vi "Parse Response for Result or Error.vi"(8 "error in":errorcluster, 10 "Response String In":string) -> (0 "error out":errorcluster, 1 "LabVIEW Error?":bool=TRUE, 2 "JSON Value out":variant)   [LabVIEW 2020, in "JSON-RPC Lib.lvlib" / "JSONRPC Client.lvclass"]
uses:
  JSONRPC Client.lvclass
  Variant JSON API/Variant JSON API.lvlib
  Variant Data Manipulation/Variant Data Manipulation.lvlib
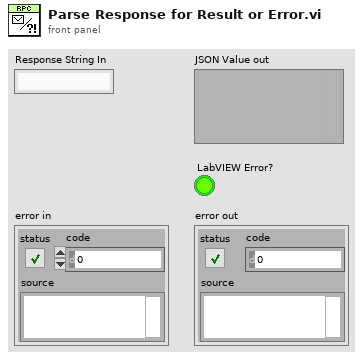
[diagram p1: front panel]
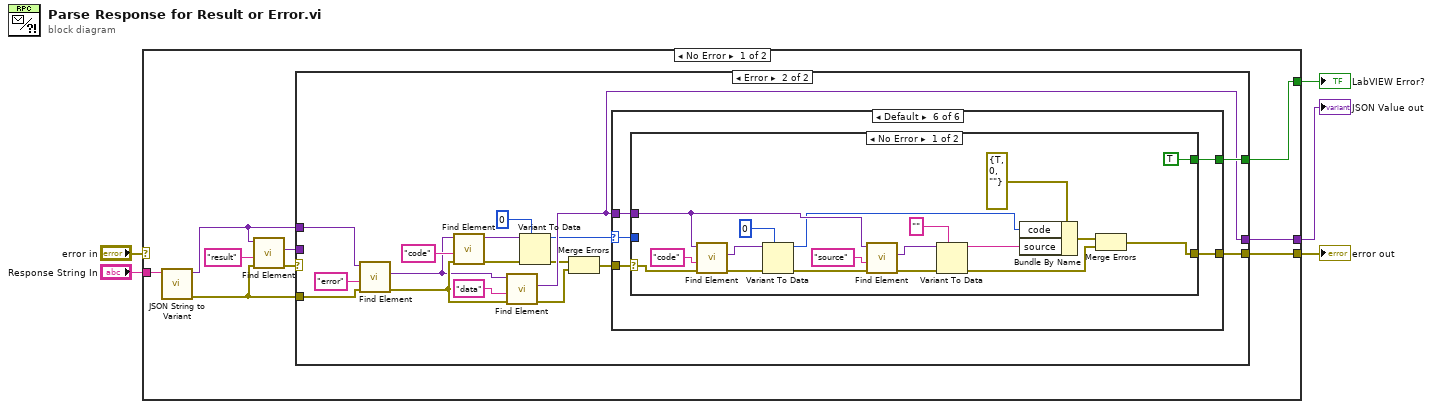
[diagram p0: block diagram]
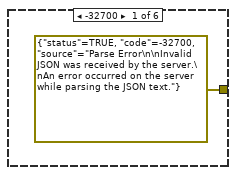
[diagram p3: hidden frame]
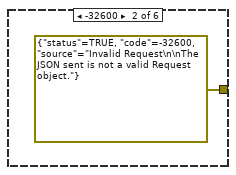
[diagram p4: hidden frame]
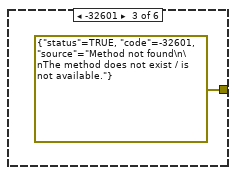
[diagram p5: hidden frame]
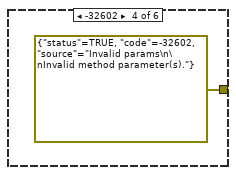
[diagram p6: hidden frame]
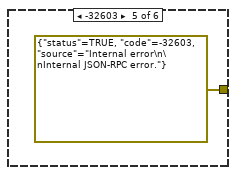
[diagram p7: hidden frame]
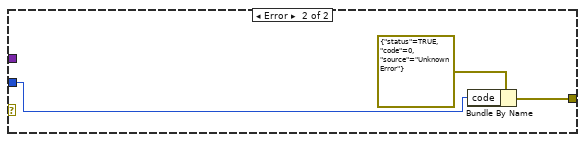
[diagram p8: hidden frame]
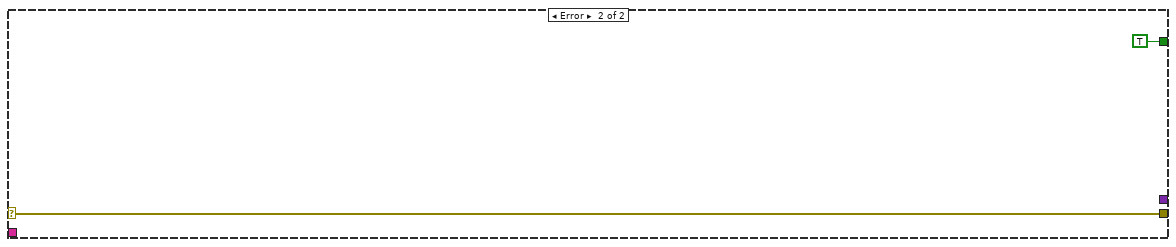
[diagram p9: hidden frame]
diagram:
  n1 = case shown="No Error" "error in" {
    selector: "error in" -> [_ w65]
    tunnel: "Response String In" -> [w11 _]
    tunnel: [w14 _] -> w1
    tunnel: [w13 w65] -> w3
    tunnel: [w12 TRUE] -> w2
    frame No Error {
      n2 = call "JSON String to Variant.vi"("JSON String"=w11) -> ("error out"=w7:errorcluster, "Variant out"=w6:variant)  [unwired: 9 in]
      n3 = call "Find Element.vi"("error in (no error)"=w7, "Name"="result" ("key"), "Variant (Cluster) in"=w6) -> ("error out"=w8:errorcluster, "element"=w9:variant)  [unwired: 4 in, 3 out]
      n4 = case shown="Error" w8 {
        selector: w8 -> [w15 _]
        tunnel: [w16 w27] -> w14
        tunnel: [w15 w33] -> w13
        tunnel: [_ w32] -> w12
        tunnel: w6 -> [_ w31]
        tunnel: w9 -> [w16 _]
        tunnel: w7 -> [_ w22]
        frame No Error {
        }
        frame Error {
          n5 = call "Find Element.vi"("error in (no error)"=w22, "Name"="error" ("key"), "Variant (Cluster) in"=w31) -> ("error out"=w26:errorcluster, "element"=w23:variant)  [unwired: 4 in, 3 out]
          n6 = call "Find Element.vi"("error in (no error)"=w26, "Name"="code" ("key"), "Variant (Cluster) in"=w23) -> ("error out"=w18:errorcluster, "Variant (Cluster) out"=w20:variant)  [unwired: 4 in, 3 out]
          n7 = call "Find Element.vi"("error in (no error)"=w26, "Name"="data" ("key"), "Variant (Cluster) in"=w23) -> ("error out"=w25:errorcluster, "element"=w27:variant)  [unwired: 4 in, 3 out]
          n8 = Variant To Data(error in=w18, type=0 ("32bit integer"), Variant=w20) -> (data=w19:i32, error out=w17:errorcluster)
          n9 = Merge Errors(w17, w25) -> (w24:errorcluster)
          n10 = case shown="Default" w19 {
            selector: w19 -> [_ _ _ _ _ w41]
            tunnel: [errorcluster {"status"=TRUE, "code"=-32700, "source"="Parse Error\n\nInvalid JSON was received by the server.\nAn error occurred on the server while parsing the JSON text."} ("error constant") errorcluster {"status"=TRUE, "code"=-32600, "source"="Invalid Request\n\nThe JSON sent is not a valid Request object."} ("error constant") errorcluster {"status"=TRUE, "code"=-32601, "source"="Method not found\n\nThe method does not exist / is not available."} ("error constant") errorcluster {"status"=TRUE, "code"=-32602, "source"="Invalid params\n\nInvalid method parameter(s)."} ("error constant") errorcluster {"status"=TRUE, "code"=-32603, "source"="Internal error\n\nInternal JSON-RPC error."} ("error constant") w43] -> w33
            tunnel: w27 -> [_ _ _ _ _ w42]
            tunnel: [_ _ _ _ _ w40] -> w32
            tunnel: w24 -> [_ _ _ _ _ w39]
            frame -32700 {
            }
            frame -32600 {
            }
            frame -32601 {
            }
            frame -32602 {
            }
            frame -32603 {
            }
            frame Default {
              n11 = case shown="No Error" w39 {
                selector: w39 -> [w46 _]
                tunnel: [w56 w62] -> w43
                tunnel: w42 -> [w55 _]
                tunnel: w41 -> [_ w63]
                tunnel: [TRUE _] -> w40
                frame No Error {
                  n12 = call "Find Element.vi"("error in (no error)"=w46, "Name"="code" ("key"), "Variant (Cluster) in"=w55) -> ("error out"=w47:errorcluster, "element"=w52:variant)  [unwired: 4 in, 3 out]
                  n13 = Variant To Data(error in=w47, type=0 ("code"), Variant=w52) -> (data=w51:i32, error out=w45:errorcluster)
                  n14 = call "Find Element.vi"("error in (no error)"=w45, "Name"="source" ("Parameter Name"), "Variant (Cluster) in"=w55) -> ("error out"=w44:errorcluster, "element"=w50:variant)  [unwired: 4 in, 3 out]
                  n15 = Variant To Data(error in=w44, type="" ("source"), Variant=w50) -> (data=w49:string, error out=w48:errorcluster)
                  n16 = Bundle By Name(cluster=errorcluster {"status"=TRUE, "code"=0, "source"=""} ("error constant"), "code"=w51, "source"=w49) -> (w57:errorcluster)
                  n17 = Merge Errors(w57, w48) -> (w56:errorcluster)
                }
                frame Error {
                  n18 = Bundle By Name(cluster=errorcluster {"status"=TRUE, "code"=0, "source"="Unknown Error"} ("error constant"), "code"=w63) -> (w62:errorcluster)
                }
              }
            }
          }
        }
      }
    }
    frame Error {
    }
  }
  "error out" <- w3
  "JSON Value out" <- w1
  "LabVIEW Error?" <- w2
